vi "Switch Connect.vi"(7 "Channel Specs":string[][](array[string]), 8 "error in (no error)":errorcluster, 9 "Channel Index":i32=6, 10 "IVI Specifications":string[][](array[string]), 11 "Switch Refs":refnum<k15>[](array[refnum])) -> (0 "error out":errorcluster, 2 "Channels Connected":string[](array[string]), 3 "Refs Connected":refnum<k15>[](array[refnum]))   [LabVIEW 2019]
uses:
  <instrlib>/niSwitch/niSwitch.llb/niSwitch Connect Channels (Multiple).vi
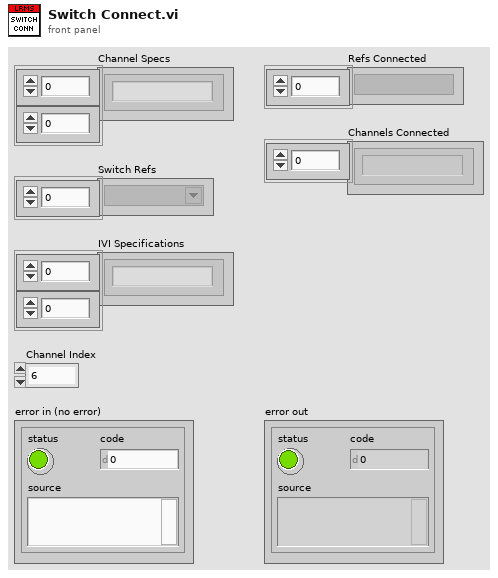
[diagram p1: front panel]
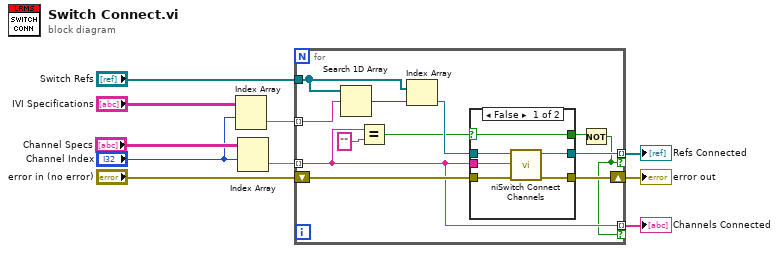
[diagram p0: block diagram]
diagram:
  n1 = Index Array(array="IVI Specifications", index (row)="Channel Index") -> (element=w1:string[])  [unwired: 1 in]
  n2 = Index Array(array="Channel Specs", index (row)="Channel Index") -> (element=w8:string[])  [unwired: 1 in]
  n3 = for {
    tunnel: w1 -> [w22] mode=indexing
    tunnel: "Switch Refs" -> [w14]
    tunnel: w8 -> [w12] mode=indexing
    tunnel: [w18] -> w9 mode=indexing if=w11
    shift-right: [w17] -> w7
    shift-left: "error in (no error)" -> [w19]
    tunnel: [w12] -> w10 mode=indexing if=w11
    n4 = Search 1D Array(1D array=w14, element=w22) -> (index of element=w21:i32)  [unwired: 1 in]
    n5 = Equal?(x=w12, y="") -> (x = y?=w15:bool)
    n6 = Index Array(array=w14, index=w21) -> (element=w20:refnum<k15>)
    n7 = case shown="False" w15 {
      selector: w15 -> [w23 w29]
      tunnel: w20 -> [w28 w31]
      tunnel: w19 -> [w27 w30]
      tunnel: [w26 w31] -> w18
      tunnel: [w25 w30] -> w17
      tunnel: w12 -> [w24 _]
      tunnel: [w23 w29] -> w13
      frame False {
        n8 = call-poly <instrlib>:"niSwitch Connect Channels.vi"("error in (no error)"=w27, "connection list"=w24, "instrument handle"=w28) -> ("error out"=w25:errorcluster, "instrument handle out"=w26:refnum<k15>)  [unwired: 7 in]
      }
      frame True {
      }
    }
    n9 = Not(x=w13) -> (.not. x?=w11:bool)
  }
  "Channels Connected" <- w10
  "Refs Connected" <- w9
  "error out" <- w7
